vi "Write Channel info.vi"(8 "error in":errorcluster, 10 "channel info":T1, 11 "channel in":refnum<class "_Channel.lvclass">) -> (0 "error out":errorcluster, 3 "channel out":refnum<class "_Channel.lvclass">)   [LabVIEW 2013, in "_Channel.lvclass"]
uses:
  _Channel.lvclass
  cRIO Repo/ChannelData.ctl
  _Channel.lvclass/_Channel.ctl
  cRIO Repo/_cRIORepo.lvclass
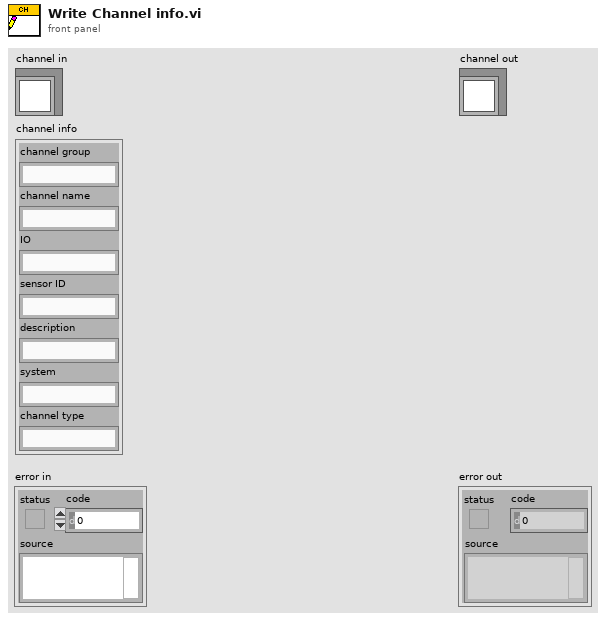
[diagram p1: front panel]
types:
  T1 = typedef "_cRIORepo.lvclass/ChannelData.ctl" = cluster{"channel group":string, "channel name":string, "IO ":string, "sensor ID":string, "description":string, "system":string, "channel type":string}
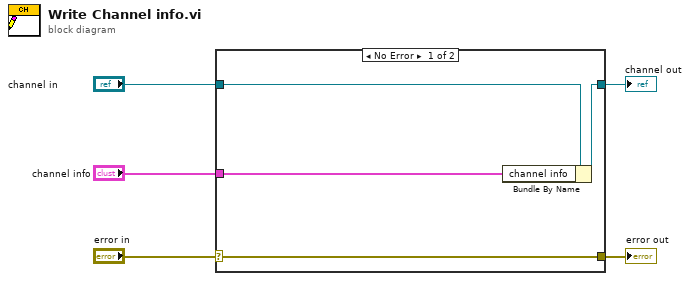
[diagram p0: block diagram]
diagram:
  n1 = case shown="No Error" "error in" {
    selector: "error in" -> [w9 w10]
    tunnel: [w9 w10] -> w4
    tunnel: [w7 w11] -> w2
    tunnel: "channel in" -> [w8 w11]
    tunnel: "channel info" -> [w6 _]
    frame No Error {
      n2 = Bundle By Name(cluster=w8, "channel info"=w6) -> (w7:refnum<class "_Channel.lvclass">)
    }
    frame Error {
    }
  }
  "error out" <- w4
  "channel out" <- w2
